vi "Write String Array Units.vi"(5 "Total_1":dbl, 6 "Pilot Rate (BTU/hr)":dbl=600.0, 7 "HHV_1":dbl, 8 "Error In":errorcluster, 9 "Gross Heating Value, Vol (Real, Dry)":dbl=1000.0 min=900.0 max=2600.0 step=1.0, 11 "Gas Data":T1) -> (0 "Error Out":errorcluster, 2 "Burner ON?":bool, 3 "String Data":string[][](array[string]))   [LabVIEW 2020]
uses:
  Modbus/Modbus Gas Meter Data.ctl
  Data Cluster.ctl
  Units of Measure.ctl
panel:
  in  "Header Array Debug":string[](array[string])=["Time Stamp", "Absolute Pressure", "Gauge/Diff. Pressure", "BarometricPressure", "Temperature", "Uncorrected", "Corrected", "Totalizer", "Tot. Timer", "Tot. Avg. Flow", "Tot. Peak Flow", "Gas Selected"]
  # "Totalizer Timer"
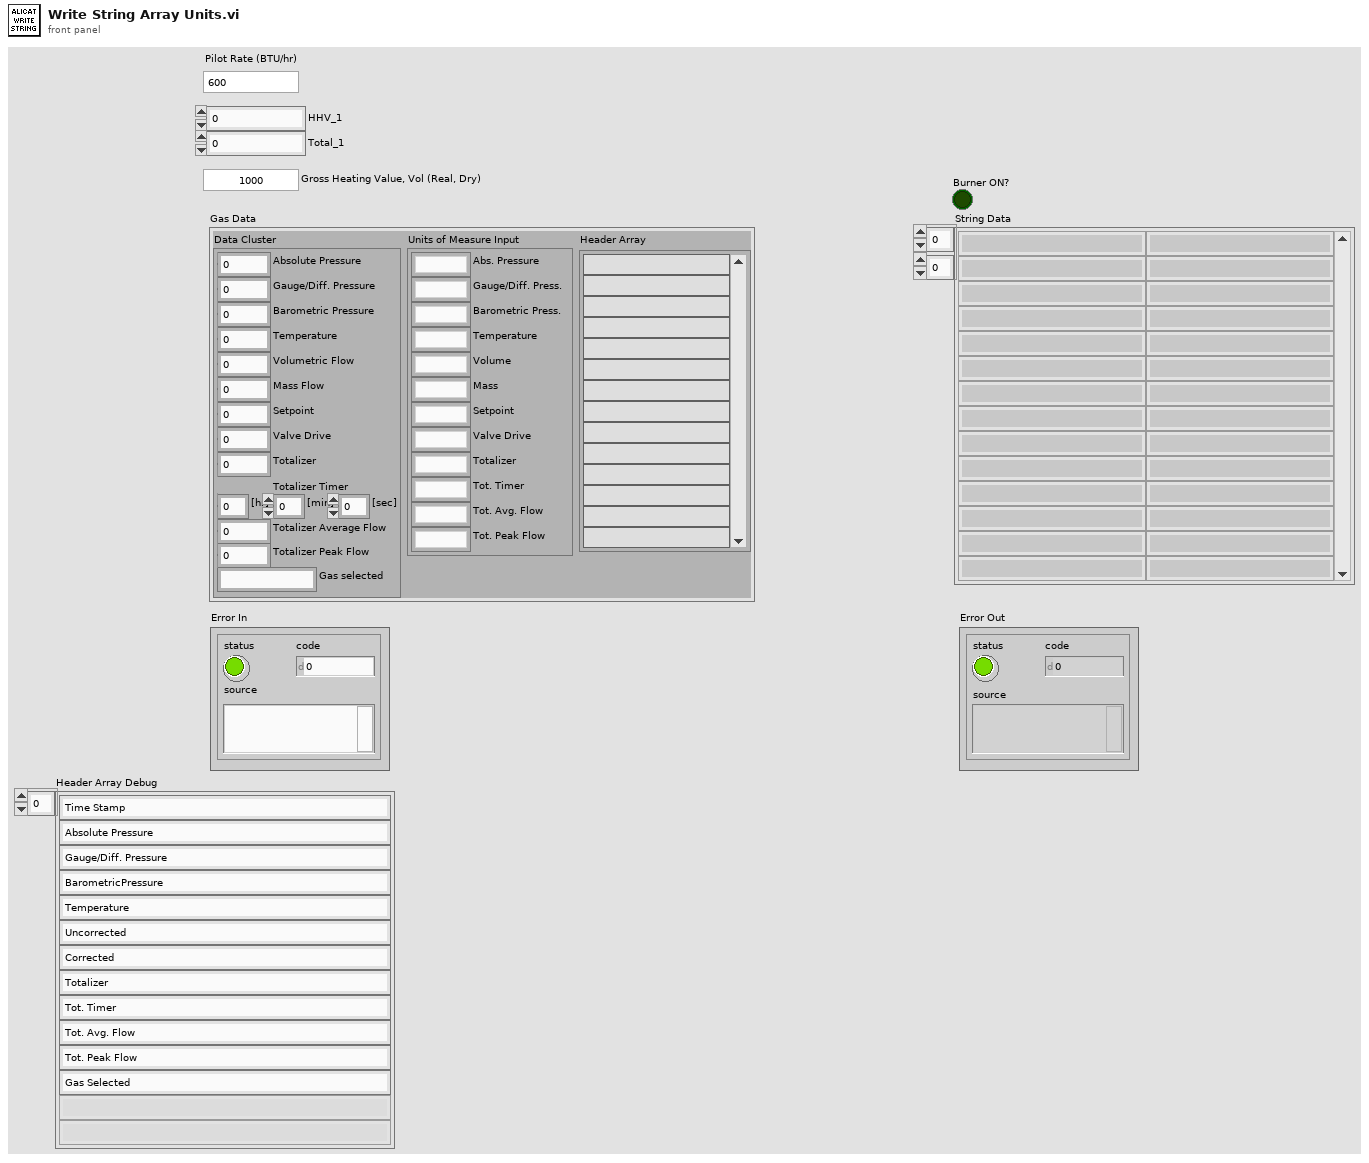
[diagram p1: front panel]
types:
  T1 = typedef "Modbus Gas Meter Data.ctl" = cluster{"Data Cluster":T2, "Units of Measure Input":T3, "Header Array":string[]}
  T2 = typedef "Data Cluster.ctl" = cluster{"Absolute Pressure":dbl, "Gauge/Diff. Pressure":dbl, "Barometric Pressure":dbl, "Temperature":dbl, "Volumetric Flow":dbl, "Mass Flow":dbl, "Setpoint":dbl, "Valve Drive":dbl, "Totalizer":dbl, "[hr]":dbl, "[min]":dbl, "[sec]":dbl, "Totalizer Average Flow":dbl, "Totalizer Peak Flow":dbl, "Gas selected":string}
  T3 = typedef "Units of Measure.ctl" = cluster{"Abs. Pressure":string, "Gauge/Diff. Press.":string, "Barometric Press.":string, "Temperature":string, "Volume":string, "Mass":string, "Setpoint":string, "Valve Drive":string, "Totalizer":string, "Tot. Timer":string, "Tot. Avg. Flow":string, "Tot. Peak Flow":string}
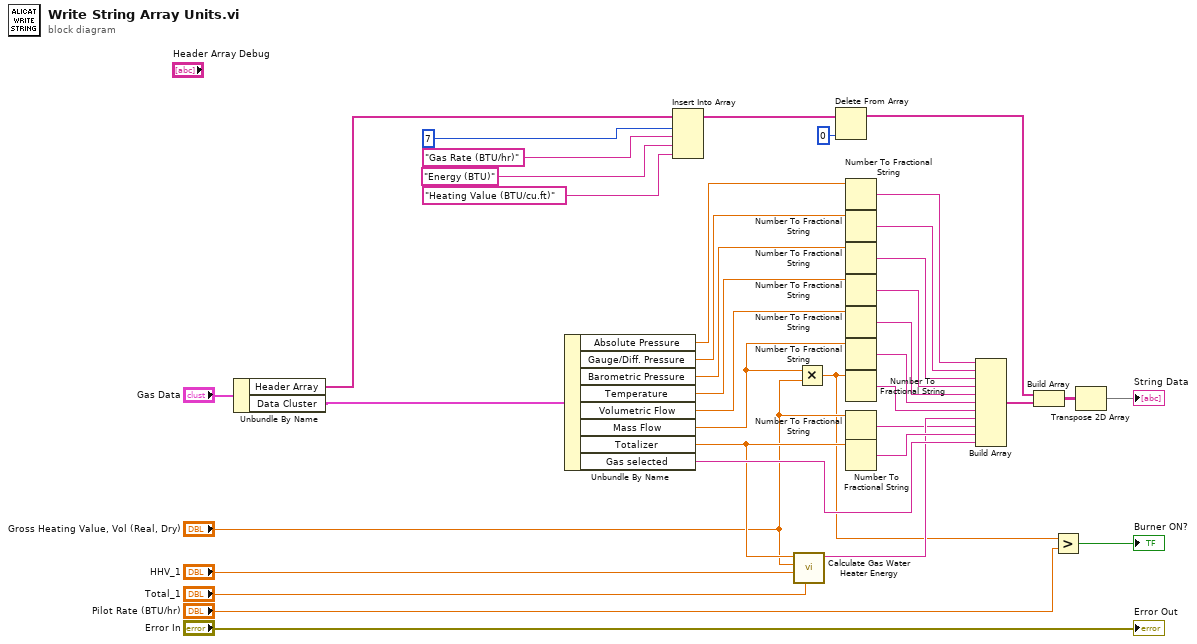
[diagram p0: block diagram]
diagram:
  n1 = Unbundle By Name("Gas Data") -> ("Header Array"=w5:string[], "Data Cluster"=w4:T2)
  n2 = Unbundle By Name(w4) -> ("Absolute Pressure"=w32:dbl, "Gauge/Diff. Pressure"=w33:dbl, "Barometric Pressure"=w34:dbl, "Temperature"=w35:dbl, "Volumetric Flow"=w36:dbl, "Mass Flow"=w21:dbl, "Totalizer"=w15:dbl, "Gas selected"=w25:string)
  n3 = Insert Into Array(array=w5, index=7, new element #1="Gas Rate (BTU/hr)" ("new element/subarray"), new element #2="Energy (BTU)" ("new element/subarray"), new element #3="Heating Value (BTU/cu.ft)" ("new element/subarray")) -> (w17:string[])
  n4 = call "Calculate Gas Water Heater Energy.vi"("Total_1"="Total_1", "HHV_1"="HHV_1", "Gross Heating Value, Vol (Real, Dry) in"="Gross Heating Value, Vol (Real, Dry)", "Totalizer"=w15) -> ("Total Energy"=w11:string)  [unwired: 4 in, 3 out]
  n5 = Multiply(x=w21, y="Gross Heating Value, Vol (Real, Dry)") -> (x*y=w1:dbl)
  n6 = Delete From Array(array=w17, index=0) -> (array with subset deleted=w10:string[])  [unwired: 1 in, 1 out]
  n7 = Number To Fractional String(number=w32) -> (F-format string=w31:string)  [unwired: 3 in]
  n8 = Number To Fractional String(number=w33) -> (F-format string=w30:string)  [unwired: 3 in]
  n9 = Number To Fractional String(number=w34) -> (F-format string=w29:string)  [unwired: 3 in]
  n10 = Number To Fractional String(number=w35) -> (F-format string=w28:string)  [unwired: 3 in]
  n11 = Number To Fractional String(number=w36) -> (F-format string=w27:string)  [unwired: 3 in]
  n12 = Number To Fractional String(number=w21) -> (F-format string=w26:string)  [unwired: 3 in]
  n13 = Number To Fractional String(number=w1) -> (F-format string=w20:string)  [unwired: 3 in]
  n14 = Number To Fractional String(number="Gross Heating Value, Vol (Real, Dry)") -> (F-format string=w7:string)  [unwired: 3 in]
  n15 = Number To Fractional String(number=w15) -> (F-format string=w16:string)  [unwired: 3 in]
  n16 = Build Array(w31, w30, w29, w28, w27, w26, w20, w11, w7, w16, w25) -> (w24:string[])
  n17 = Build Array(w10, w24) -> (w37:string[][])
  n18 = Greater?(x=w1, y="Pilot Rate (BTU/hr)") -> (0:→"Burner ON?":bool)
  n19 = Transpose 2D Array(2D array=w37) -> (transposed array=→"String Data":string[][])
  "Error Out" <- "Error In"
